vi "Scan Service Level.vi"(4 "Days Open Prio Threshold":dbl=1.0, 5 "English Tags":string[](array[string])=["\\[ENG\\]"], 6 "Include High Priority?":bool=TRUE, 7 "Premier Levels Keywords":string[](array[string])=["Premier", "SRLLEASE", "VLA"], 8 "error in (no error)":errorcluster, 11 "Array in":T1(array[cluster])) -> (0 "error out":errorcluster, 3 "Array out":T1(array[cluster]))   [LabVIEW 2017, in "Client.lvlib" / "ParserSorter.lvlib"]
doc: "Determine SR Priority"
uses:
  ParserSorter.lvlib
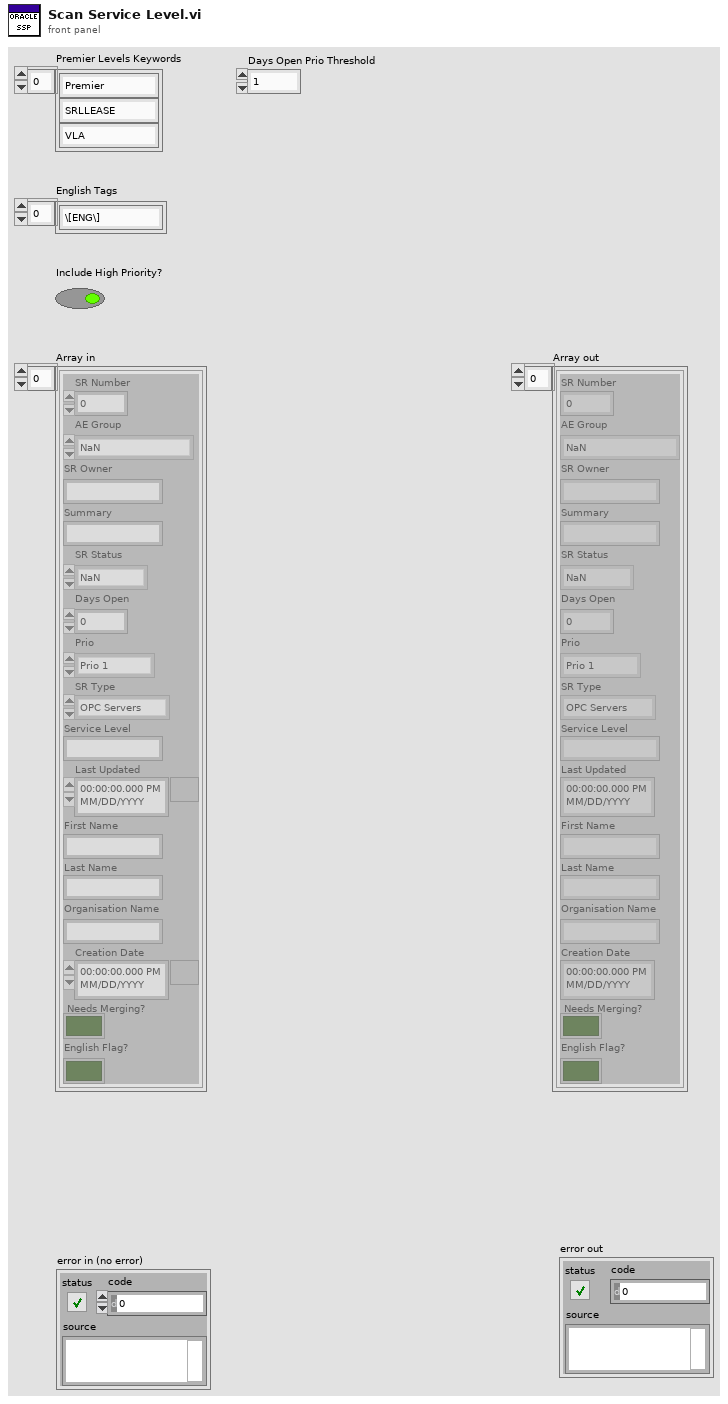
[diagram p1: front panel]
types:
  T1 = cluster{"SR Number":i64, "AE Group":enum32{"NaN", "AE-Germany", "AE-Poland", "AE-Switzerland", "AE-Czech Republic", "AE-Hungary", "AE-Romania", "AE-Slovakia", "AE-Slovenia"}, "SR Owner":string, "Summary":string, "SR Status":enum32{"NaN", "Caller Abandoned", "Created in Error", "Declined to Purchase Support", "Expired", "Forum Resolved AE", "Forum Resolved Customer", "IN WORK", "IN WORK Collab with AES", "IN WORK Collab with PSE", "IN WORK Collab with SE", "IN WORK Escalation", "IN WORK Customer Added Note", "Open", "Potentially Resolved", "POC Resolved", "Resolved", "RMA Waiting on Customer", "RMA Open", "RMA In Progress", "RMA Closed - DOA", "RMA Closed", "RMA Approved for Return", "Project Complete", "Presumed Resolved", "IN WORK Wait on Customer"}, "Days Open":dbl, "Prio":enum16{"Prio 1", "Prio 2", "Prio 3", "Prio 4"}, "SR Type":enum32{"NaN", "ATE Core Configurations (BYOATE)", "Activation", "BioBench", "CAN", "CM C Series", "Calibration", "Consulting Services", "CounterTimer", "DAQExpress", "DASYLab", "DIAdem", "DMM", "DSA HW", "Digital_IO", "FIRST (NIC Only)", "FieldBus", "FieldPoint", "Functional Savety", "GATI", "GPIB", "HMI and Industrial PCs", "HiQ", "HighSpeedDigital_IO", "IMAQ", "IOTech Vibration", "Industrial Communications", "InsightCM", "LV", "LV CD&Sim", "LV Comms", "LV Controls Add-Ons", "LV Embedded", "LV MathScript RT", "LV NXG", "LV NXT", "LVDSC", "LVFPGA", "LVPDA and LV Touch Panel", "LVRT", "LabWindows_CVI", "Lookout", "MATRIXx", "MStudioDotNet", "MStudioVisualBasic", "MStudioVisualC", "Measure (Legacy)", "Motion", "MultifunctionDAQ", "Multimedia Test HW/SW", "Multisim (EWB)", "NI Update Service", "OPC Servers", "Optical (OSI)", "PXI Controllers, Chassis, MXI", "PXI Timing and Sync", "Power Supplies and SMUs", "Powertrain Controls", "RAID", "RF", "RF Software", "RIO", "SC Express", "SCC", "SCXI", "SPEEDY-33 (Hyperception)", "STS", "ScopeDigitizers", "Serial", "Signal Sources", "SignalCondOther", "SignalExpress", "Software Defined Intruments", "Sound and Vibration SW", "Switch Executive", "Switches", "TestStand", "USRP", "Ultiboard (EWB)", "VBench", "VI Logger", "VXI_MXI", "VeriStand", "VisionSW", "VolumeLicenseMgr", "WSN", "Web UI Builder", "myRIO"}, "Service Level":string, "Last Updated":timestamp, "First Name":string, "Last Name":string, "Organisation Name":string, "Creation Date":timestamp, "Needs Merging?":bool, "English Flag?":bool}[]
  T2 = cluster{"SR Number":i64, "AE Group":enum32{"NaN", "AE-Germany", "AE-Poland", "AE-Switzerland", "AE-Czech Republic", "AE-Hungary", "AE-Romania", "AE-Slovakia", "AE-Slovenia"}, "SR Owner":string, "Summary":string, "SR Status":enum32{"NaN", "Caller Abandoned", "Created in Error", "Declined to Purchase Support", "Expired", "Forum Resolved AE", "Forum Resolved Customer", "IN WORK", "IN WORK Collab with AES", "IN WORK Collab with PSE", "IN WORK Collab with SE", "IN WORK Escalation", "IN WORK Customer Added Note", "Open", "Potentially Resolved", "POC Resolved", "Resolved", "RMA Waiting on Customer", "RMA Open", "RMA In Progress", "RMA Closed - DOA", "RMA Closed", "RMA Approved for Return", "Project Complete", "Presumed Resolved", "IN WORK Wait on Customer"}, "Days Open":dbl, "Prio":enum16{"Prio 1", "Prio 2", "Prio 3", "Prio 4"}, "SR Type":enum32{"NaN", "ATE Core Configurations (BYOATE)", "Activation", "BioBench", "CAN", "CM C Series", "Calibration", "Consulting Services", "CounterTimer", "DAQExpress", "DASYLab", "DIAdem", "DMM", "DSA HW", "Digital_IO", "FIRST (NIC Only)", "FieldBus", "FieldPoint", "Functional Savety", "GATI", "GPIB", "HMI and Industrial PCs", "HiQ", "HighSpeedDigital_IO", "IMAQ", "IOTech Vibration", "Industrial Communications", "InsightCM", "LV", "LV CD&Sim", "LV Comms", "LV Controls Add-Ons", "LV Embedded", "LV MathScript RT", "LV NXG", "LV NXT", "LVDSC", "LVFPGA", "LVPDA and LV Touch Panel", "LVRT", "LabWindows_CVI", "Lookout", "MATRIXx", "MStudioDotNet", "MStudioVisualBasic", "MStudioVisualC", "Measure (Legacy)", "Motion", "MultifunctionDAQ", "Multimedia Test HW/SW", "Multisim (EWB)", "NI Update Service", "OPC Servers", "Optical (OSI)", "PXI Controllers, Chassis, MXI", "PXI Timing and Sync", "Power Supplies and SMUs", "Powertrain Controls", "RAID", "RF", "RF Software", "RIO", "SC Express", "SCC", "SCXI", "SPEEDY-33 (Hyperception)", "STS", "ScopeDigitizers", "Serial", "Signal Sources", "SignalCondOther", "SignalExpress", "Software Defined Intruments", "Sound and Vibration SW", "Switch Executive", "Switches", "TestStand", "USRP", "Ultiboard (EWB)", "VBench", "VI Logger", "VXI_MXI", "VeriStand", "VisionSW", "VolumeLicenseMgr", "WSN", "Web UI Builder", "myRIO"}, "Service Level":string, "Last Updated":timestamp, "First Name":string, "Last Name":string, "Organisation Name":string, "Creation Date":timestamp, "Needs Merging?":bool, "English Flag?":bool}
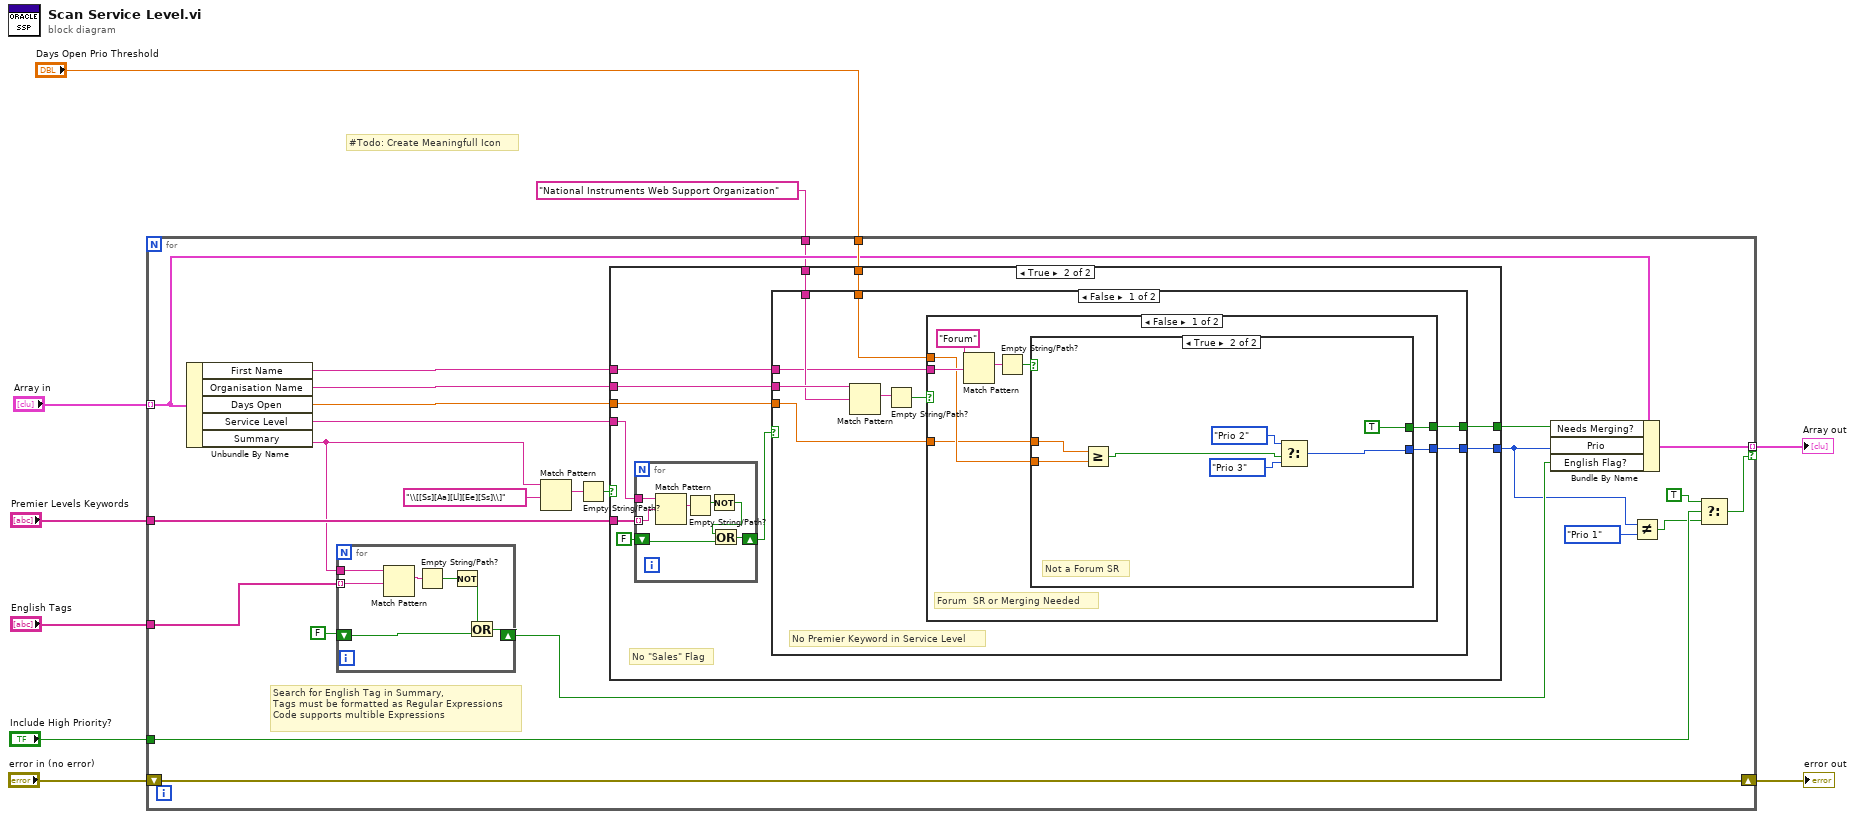
[diagram p0: block diagram]
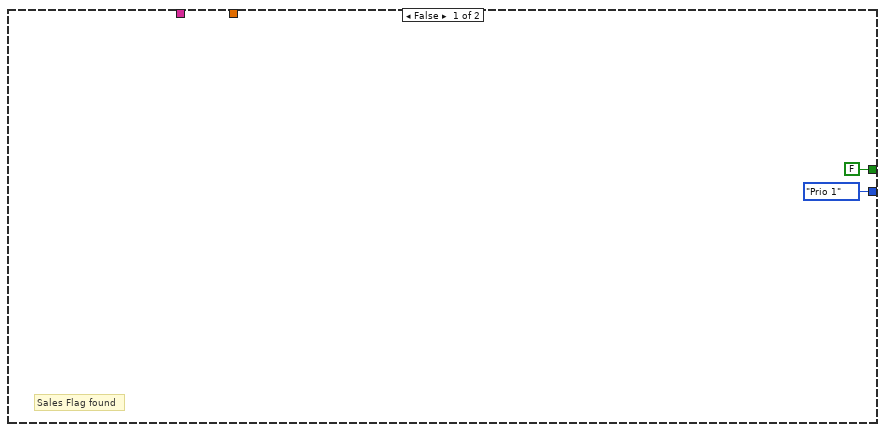
[diagram p2: hidden frame]
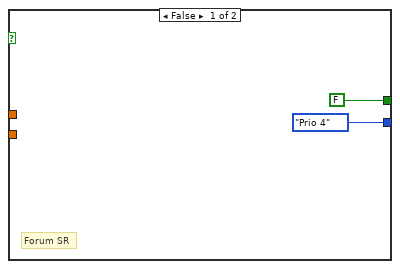
[diagram p3: hidden frame]
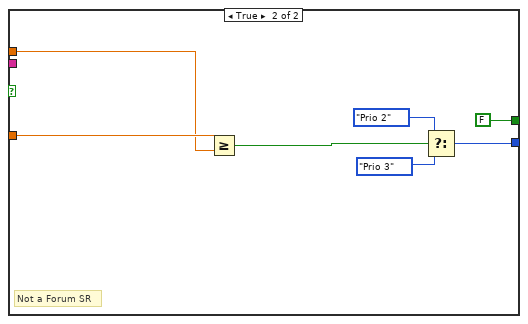
[diagram p4: hidden frame]
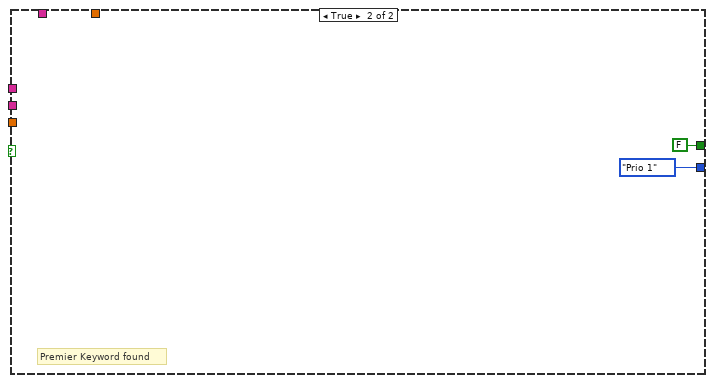
[diagram p5: hidden frame]
diagram:
  # "#Todo: Create Meaningfull Icon"
  n1 = for {
    tunnel: "Array in" -> [w25] mode=indexing
    shift-right: [w27] -> w9
    shift-left: "error in (no error)" -> [w27]
    tunnel: "Days Open Prio Threshold" -> [w26]
    tunnel: [w24] -> w3 mode=indexing if=w13
    tunnel: "Premier Levels Keywords" -> [w23]
    tunnel: "National Instruments Web Support Organization" -> [w22]
    tunnel: "English Tags" -> [w18]
    tunnel: "Include High Priority?" -> [w15]
    # "Search for English Tag in Summary, \nTags must be formatted as Regular Expressions\nCode supports multible Expressions"
    n2 = Unbundle By Name(w25) -> ("First Name"=w21:string, "Organisation Name"=w28:string, "Days Open"=w29:dbl, "Service Level"=w30:string, "Summary"=w17:string)
    n3 = for {
      tunnel: w18 -> [w40] mode=indexing
      shift-right: [w37] -> w16
      shift-left: FALSE -> [w38]
      tunnel: w17 -> [w34]
      n4 = Match Pattern(string=w34, regular expression=w40) -> (match substring=w39:string)  [unwired: 1 in, 3 out]
      n5 = Empty String/Path?(string/path=w39) -> (empty?=w36:bool)
      n6 = Not(x=w36) -> (.not. x?=w35:bool)
      n7 = Or(x=w35, y=w38) -> (x .or. y?=w37:bool)
    }
    n8 = Match Pattern(string=w17, regular expression="\\[[Ss][Aa][Ll][Ee][Ss]\\]") -> (match substring=w32:string)  [unwired: 1 in, 3 out]
    n9 = Empty String/Path?(string/path=w32) -> (empty?=w31:bool)
    n10 = case shown="True" w31 {
      tunnel: w30 -> [_ w47]
      tunnel: w29 -> [_ w53]
      tunnel: w28 -> [_ w52]
      tunnel: w26 -> [_ w51]
      tunnel: [enum16{"Prio 1", "Prio 2", "Prio 3", "Prio 4"}."Prio 1" ("f") w50] -> w12
      tunnel: w23 -> [_ w48]
      tunnel: w22 -> [_ w45]
      tunnel: w21 -> [_ w44]
      tunnel: [FALSE w43] -> w20
      frame False {
        # "Sales Flag found"
      }
      frame True {
        # "No \"Sales\" Flag"
        n11 = for {
          shift-right: [w59] -> w46
          shift-left: FALSE -> [w58]
          tunnel: w48 -> [w57] mode=indexing
          tunnel: w47 -> [w56]
          n12 = Match Pattern(string=w56, regular expression=w57) -> (match substring=w60:string)  [unwired: 1 in, 3 out]
          n13 = Empty String/Path?(string/path=w60) -> (empty?=w54:bool)
          n14 = Not(x=w54) -> (.not. x?=w55:bool)
          n15 = Or(x=w55, y=w58) -> (x .or. y?=w59:bool)
        }
        n16 = case shown="False" w46 {
          tunnel: w53 -> [w66 _]
          tunnel: w52 -> [w69 _]
          tunnel: w51 -> [w65 _]
          tunnel: [w64 enum16{"Prio 1", "Prio 2", "Prio 3", "Prio 4"}."Prio 1" ("f")] -> w50
          tunnel: w45 -> [w63 _]
          tunnel: w44 -> [w62 _]
          tunnel: [w61 FALSE] -> w43
          frame False {
            # "No Premier Keyword in Service Level"
            n17 = Match Pattern(string=w69, regular expression=w63) -> (match substring=w67:string)  [unwired: 1 in, 3 out]
            n18 = Empty String/Path?(string/path=w67) -> (empty?=w68:bool)
            n19 = case shown="False" w68 {
              tunnel: w66 -> [w73 w93]
              tunnel: w65 -> [w74 w92]
              tunnel: [w72 w88] -> w64
              tunnel: w62 -> [w76 _]
              tunnel: [w71 FALSE] -> w61
              frame False {
                # "Forum  SR or Merging Needed"
                n20 = Match Pattern(string="Forum", regular expression=w76) -> (match substring=w75:string)  [unwired: 1 in, 3 out]
                n21 = Empty String/Path?(string/path=w75) -> (empty?=w70:bool)
                n22 = case shown="True" w70 {
                  tunnel: w74 -> [_ w86]
                  tunnel: w73 -> [_ w85]
                  tunnel: [enum16{"Prio 1", "Prio 2", "Prio 3", "Prio 4"}."Prio 4" ("f") w81] -> w72
                  tunnel: [FALSE TRUE] -> w71
                  frame False {
                    # "Forum SR"
                  }
                  frame True {
                    # "Not a Forum SR"
                    n23 = Greater Or Equal?(x=w85, y=w86) -> (x >= y?=w80:bool)
                    n24 = Select(t=enum16{"Prio 1", "Prio 2", "Prio 3", "Prio 4"}."Prio 2" ("f"), s=w80, f=enum16{"Prio 1", "Prio 2", "Prio 3", "Prio 4"}."Prio 3") -> (s? t:f=w81:enum16{"Prio 1", "Prio 2", "Prio 3", "Prio 4"})
                  }
                }
              }
              frame True {
                # "Not a Forum SR"
                n25 = Greater Or Equal?(x=w93, y=w92) -> (x >= y?=w90:bool)
                n26 = Select(t=enum16{"Prio 1", "Prio 2", "Prio 3", "Prio 4"}."Prio 2" ("Prio"), s=w90, f=enum16{"Prio 1", "Prio 2", "Prio 3", "Prio 4"}."Prio 3") -> (s? t:f=w88:enum16{"Prio 1", "Prio 2", "Prio 3", "Prio 4"})
              }
            }
          }
          frame True {
            # "Premier Keyword found"
          }
        }
      }
    }
    n27 = Bundle By Name(cluster=w25, "Needs Merging?"=w20, "Prio"=w12, "English Flag?"=w16) -> (w24:T2)
    n28 = Not Equal?(x=w12, y=enum16{"Prio 1", "Prio 2", "Prio 3", "Prio 4"}."Prio 1") -> (x != y?=w10:bool)
    n29 = Select(t=TRUE, s=w15, f=w10) -> (s? t:f=w13:bool)
  }
  "error out" <- w9
  "Array out" <- w3
